vi "Autofocus Score.vi"(8 "error in (no error)":errorcluster, 10 "Frame Index":i32, 11 "Stage Controller in":refnum<class "Stage Controller.lvclass">) -> (0 "error out":errorcluster, 3 "Stage Controller out":refnum<class "Stage Controller.lvclass">)   [LabVIEW 2023, in "Stage Controller.lvlib" / "Stage Controller.lvclass"]
uses:
  Stage Controller.lvclass
  Stage Controller.lvclass/Stage Controller.ctl
  Resources/GLOBAL/GLOBAL Time-critical.vi
  <vilib>/gmath/NI_Gmath.lvlib
panel:
  out "mean value":dbl
  in  "shift length":i32=2
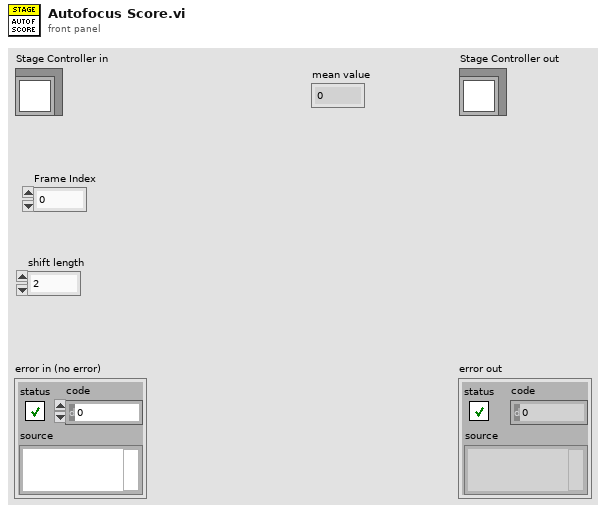
[diagram p1: front panel]
types:
  T1 = enum16{"arithmetic", "geometric", "harmonic", "trimmed", "median"}
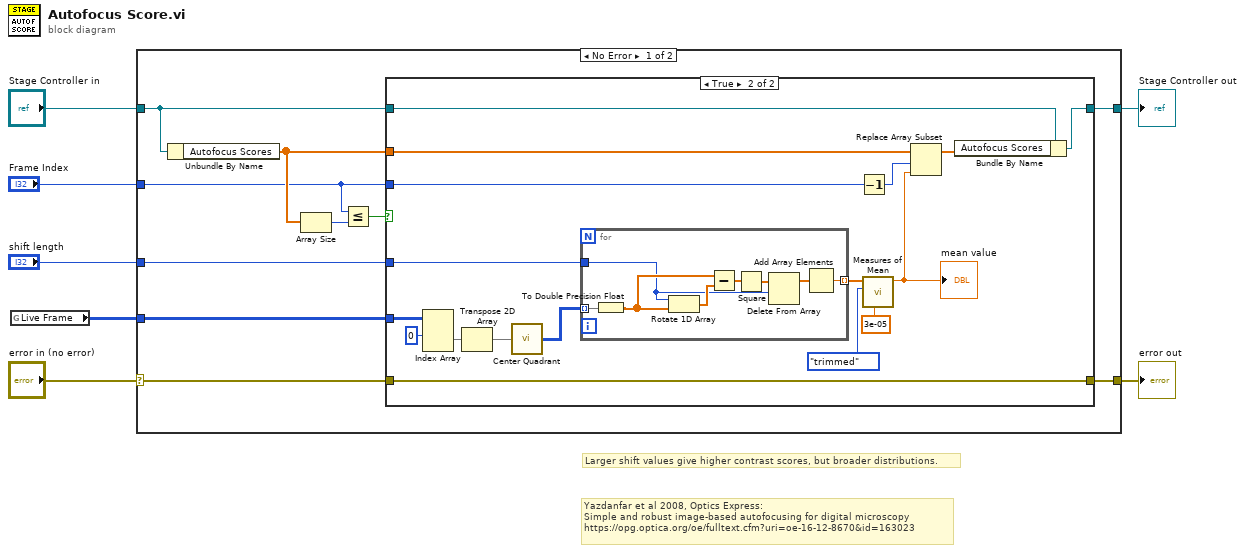
[diagram p0: block diagram]
diagram:
  # "Yazdanfar et al 2008, Optics Express:\nSimple and robust image-based autofocusing for digital microscopy \nhttps://opg.optica.org/oe/fulltext.cfm?uri=oe-16-12-8670&id=163023"
  # "Larger shift values give higher contrast scores, but broader distributions."
  n1 = global read "GLOBAL Time-critical.vi" "Live Frame"() -> (w2:u16[][][])
  n2 = case shown="No Error" "error in (no error)" {
    selector: "error in (no error)" -> [w10 w46]
    tunnel: [w9 w46] -> w6
    tunnel: [w17 w45] -> w4
    tunnel: "Stage Controller in" -> [w16 w45]
    tunnel: "shift length" -> [w15 _]
    tunnel: w2 -> [w14 _]
    tunnel: "Frame Index" -> [w8 _]
    frame No Error {
      n3 = Unbundle By Name(w16) -> ("Autofocus Scores"=w13:dbl[])
      n4 = Array Size(array=w13) -> (size(s)=w11:i32)
      n5 = Less Or Equal?(x=w8, y=w11) -> (x <= y?=w12:bool)
      n6 = case shown="True" w12 {
        tunnel: [w19 w35] -> w17
        tunnel: w16 -> [w19 w34]
        tunnel: w13 -> [_ w33]
        tunnel: w15 -> [_ w31]
        tunnel: w14 -> [_ w30]
        tunnel: w8 -> [_ w29]
        tunnel: w10 -> [w18 w22]
        tunnel: [w18 w22] -> w9
        frame False {
          # "Ignore extra frames acquired after z stack is complete."
        }
        frame True {
          n7 = Index Array(array=w30, index (dim 0)=0 ("index (page)")) -> (element=w27:u16[][])  [unwired: 2 in]
          n8 = Transpose 2D Array(2D array=w27) -> (transposed array=w21:u16[][])
          n9 = call "Center Quadrant.vi"("Array In"=w21) -> ("Center Quad"=w20:u16[][])
          n10 = for {
            tunnel: w20 -> [w41] mode=indexing
            tunnel: [w42] -> w24 mode=indexing
            tunnel: w31 -> [w37]
            # "Loop over image rows (columns?)"
            n11 = To Double Precision Float(number=w41) -> (double precision float=w40:dbl[])
            n12 = Rotate 1D Array(1:w40, 2:w37) -> (0:w43:dbl[])
            n13 = Subtract(x=w40, y=w43) -> (x-y=w44:dbl[])
            n14 = Square(x=w44) -> (x^2=w38:dbl[])
            n15 = Delete From Array(array=w38, length=w37) -> (array with subset deleted=w39:dbl[])  [unwired: 1 in, 1 out]
            n16 = Add Array Elements(numeric array=w39) -> (sum=w42:dbl)
          }
          n17 = Decrement(x=w29) -> (x-1=w28:i32)
          n18 = call <vilib>:"Measures of Mean.vi"("percent (trim)"=3e-05, "type"=T1."trimmed", "x array"=w24) -> ("mean value"=w23:dbl)  [unwired: 7 in, 1 out]
          "mean value" <- w23
          n19 = Replace Array Subset(array=w33, new element=w23, index=w28) -> (w36:dbl[])
          n20 = Bundle By Name(cluster=w34, "Autofocus Scores"=w36) -> (w35:refnum<class "Stage Controller.lvclass">)
        }
      }
    }
    frame Error {
    }
  }
  "error out" <- w6
  "Stage Controller out" <- w4
